vi "HDF5_Write_UPS_Record.vi"(0 "HealthRefs":T2 {"TimeStamp_dset" format="%.0x"; "TimeString_dset" format="%.0x"; "%_dset" format="%.0x"; "W_dset" format="%.0x"; "Hz_dset" format="%.0x"; "A_dset" format="%.0x"; "V_dset" format="%.0x"; "Group_ref" format="%.0x"}, 7 "UPS":T1, 11 "error in":errorcluster) -> (15 "error out":errorcluster)   [LabVIEW 2018]
doc: "Write a single Noise<x> record with timestamp:\nNoise1\n NoiseInfo - cluster with Timestamp and other metadata for this record\n SummdSpectrum - 1024 element Double array (waveform)"
uses:
  <vilib>/addons/h5labview2/dataset/H5D.lvlib
  <vilib>/addons/h5labview2/dataset/H5Dwrite.llb/H5Dwrite.xnode
  <vilib>/addons/h5labview2/space/H5S.lvlib
  <vilib>/addons/h5labview2/base/H5Equery.vi
  <vilib>/addons/h5labview2/base/lib_path.vi
  <vilib>/addons/h5labview2/base/hid_t_renamed.ctl
  UPS_refs.ctl
  Controls/Clusts/UPS_Status_Clust.ctl
  <vilib>/addons/h5labview2/base/hid_t.ctl
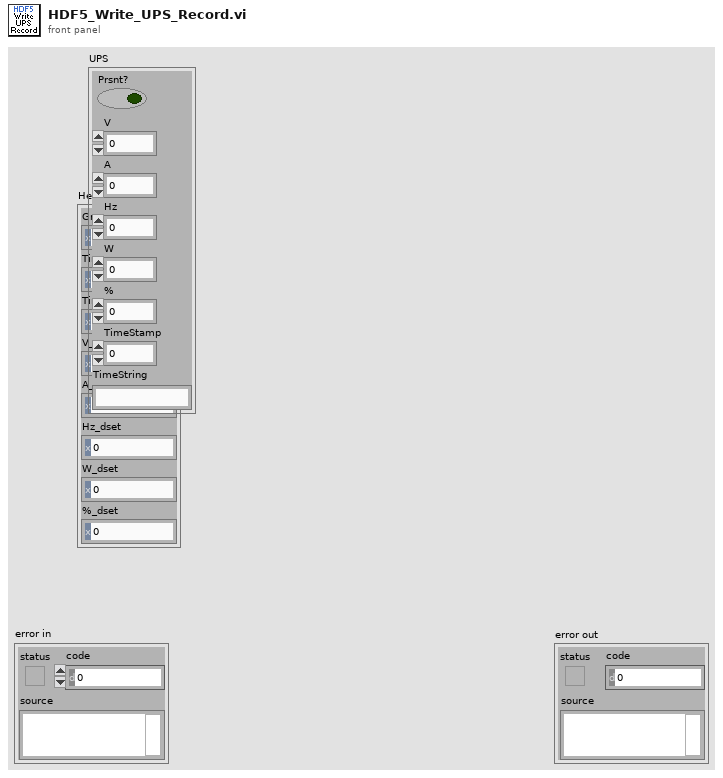
[diagram p1: front panel]
types:
  T1 = typedef "UPS_Status_Clust.ctl" = cluster{"Prsnt?":bool, "V":dbl, "A":dbl, "Hz":dbl, "W":dbl, "%":dbl, "TimeStamp":dbl, "TimeString":string}
  T2 = typedef "UPS_refs.ctl" = cluster{"Group_ref":T3, "TimeString_dset":T3, "TimeStamp_dset":T3, "V_dset":T3, "A_dset":T3, "Hz_dset":T3, "W_dset":T3, "%_dset":T3}
  T3 = typedef "hid_t.ctl" = i32
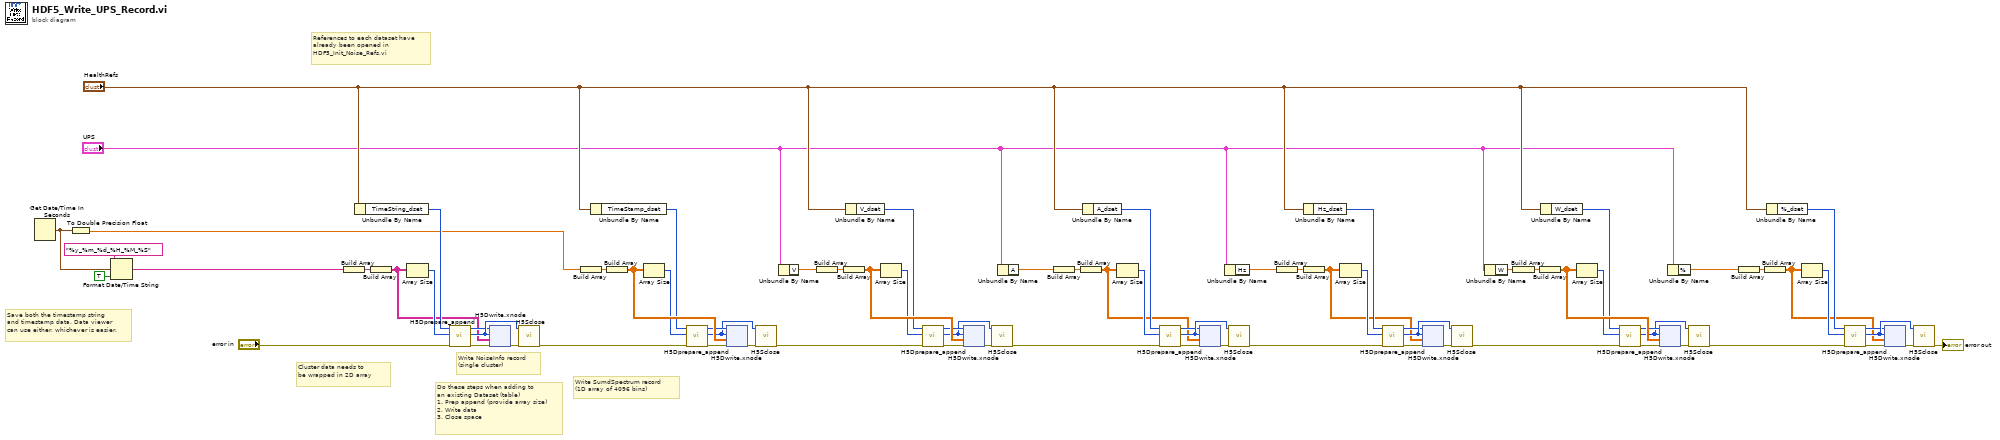
[diagram p0: block diagram]
diagram:
  # "Save both the timestamp string\nand timestamp data. Data viewer\ncan use either, whichever is easier."
  # "Cluster data needs to \nbe wrapped in 2D array"
  # "References to each dataset have \nalready been opened in \nHDF5_Init_Noise_Refs.vi"
  # "Do these steps when adding to \nan existing Dataset (table)\n1. Prep append (provide array size)\n2. Write data\n3. Close space"
  # "Write SumdSpectrum record\n(1D array of 4096 bins)"
  # "Write NoiseInfo record\n(single cluster)"
  n1 = Get Date/Time In Seconds() -> (seconds since 1Jan1904=w67:timestamp)
  n2 = To Double Precision Float(number=w67) -> (double precision float=w55:dbl)
  n3 = Format Date/Time String(time format string (%c)="%y_%m_%d_%H_%M_%S", seconds (now)=w67, UTC format=TRUE) -> (date/time string=w64:string)
  n4 = Build Array(w64) -> (w71:string[])
  n5 = Unbundle By Name("HealthRefs") -> ("TimeString_dset"=w70:T3)
  n6 = Build Array(w71) -> (w66:string[][])
  n7 = Array Size(array=w66) -> (size(s)=w69:i32[])
  n8 = call <vilib>:"H5Dprepare_append.vi"("error in (no error)"="error in", "append dims"=w69, "dset in"=w70) -> ("error out"=w76:errorcluster, "space out"=w74:T3, "dset out"=w73:T3)  [unwired: 5 in, 1 out]
  n9 = xnode "H5Dwrite.xnode"("error in (no error)"=w76, "data"=w66, "file space"=w74, "ref in"=w73) -> ("error out"=w75:errorcluster)  [unwired: 3 in, 2 out]
  n10 = call <vilib>:"H5Sclose.vi"("error in (no error)"=w75, "space in"=w74) -> ("error out"=w54:errorcluster)  [unwired: 9 in]
  n11 = Build Array(w55) -> (w60:dbl[])
  n12 = Unbundle By Name("HealthRefs") -> ("TimeStamp_dset"=w61:T3)
  n13 = Build Array(w60) -> (w63:dbl[][])
  n14 = Array Size(array=w63) -> (size(s)=w62:i32[])
  n15 = call <vilib>:"H5Dprepare_append.vi"("error in (no error)"=w54, "append dims"=w62, "dset in"=w61) -> ("error out"=w56:errorcluster, "space out"=w58:T3, "dset out"=w59:T3)  [unwired: 5 in, 1 out]
  n16 = xnode "H5Dwrite.xnode"("error in (no error)"=w56, "data"=w63, "file space"=w58, "ref in"=w59) -> ("error out"=w57:errorcluster)  [unwired: 3 in, 2 out]
  n17 = call <vilib>:"H5Sclose.vi"("error in (no error)"=w57, "space in"=w58) -> ("error out"=w9:errorcluster)  [unwired: 9 in]
  n18 = Unbundle By Name("UPS") -> ("V"=w7:dbl)
  n19 = Build Array(w7) -> (w41:dbl[])
  n20 = Build Array(w41) -> (w44:dbl[][])
  n21 = Unbundle By Name("HealthRefs") -> ("V_dset"=w42:T3)
  n22 = Array Size(array=w44) -> (size(s)=w43:i32[])
  n23 = call <vilib>:"H5Dprepare_append.vi"("error in (no error)"=w9, "append dims"=w43, "dset in"=w42) -> ("error out"=w37:errorcluster, "space out"=w39:T3, "dset out"=w40:T3)  [unwired: 5 in, 1 out]
  n24 = xnode "H5Dwrite.xnode"("error in (no error)"=w37, "data"=w44, "file space"=w39, "ref in"=w40) -> ("error out"=w38:errorcluster)  [unwired: 3 in, 2 out]
  n25 = call <vilib>:"H5Sclose.vi"("error in (no error)"=w38, "space in"=w39) -> ("error out"=w53:errorcluster)  [unwired: 9 in]
  n26 = Unbundle By Name("UPS") -> ("A"=w6:dbl)
  n27 = Build Array(w6) -> (w48:dbl[])
  n28 = Build Array(w48) -> (w45:dbl[][])
  n29 = Unbundle By Name("HealthRefs") -> ("A_dset"=w47:T3)
  n30 = Array Size(array=w45) -> (size(s)=w46:i32[])
  n31 = call <vilib>:"H5Dprepare_append.vi"("error in (no error)"=w53, "append dims"=w46, "dset in"=w47) -> ("error out"=w52:errorcluster, "space out"=w50:T3, "dset out"=w49:T3)  [unwired: 5 in, 1 out]
  n32 = xnode "H5Dwrite.xnode"("error in (no error)"=w52, "data"=w45, "file space"=w50, "ref in"=w49) -> ("error out"=w51:errorcluster)  [unwired: 3 in, 2 out]
  n33 = Unbundle By Name("UPS") -> ("Hz"=w5:dbl)
  n34 = call <vilib>:"H5Sclose.vi"("error in (no error)"=w51, "space in"=w50) -> ("error out"=w10:errorcluster)  [unwired: 9 in]
  n35 = Build Array(w5) -> (w32:dbl[])
  n36 = Unbundle By Name("HealthRefs") -> ("Hz_dset"=w31:T3)
  n37 = Build Array(w32) -> (w29:dbl[][])
  n38 = Array Size(array=w29) -> (size(s)=w30:i32[])
  n39 = call <vilib>:"H5Dprepare_append.vi"("error in (no error)"=w10, "append dims"=w30, "dset in"=w31) -> ("error out"=w36:errorcluster, "space out"=w34:T3, "dset out"=w33:T3)  [unwired: 5 in, 1 out]
  n40 = xnode "H5Dwrite.xnode"("error in (no error)"=w36, "data"=w29, "file space"=w34, "ref in"=w33) -> ("error out"=w35:errorcluster)  [unwired: 3 in, 2 out]
  n41 = call <vilib>:"H5Sclose.vi"("error in (no error)"=w35, "space in"=w34) -> ("error out"=w20:errorcluster)  [unwired: 9 in]
  n42 = Unbundle By Name("UPS") -> ("W"=w2:dbl)
  n43 = Build Array(w2) -> (w25:dbl[])
  n44 = Build Array(w25) -> (w28:dbl[][])
  n45 = Unbundle By Name("HealthRefs") -> ("W_dset"=w26:T3)
  n46 = Array Size(array=w28) -> (size(s)=w27:i32[])
  n47 = call <vilib>:"H5Dprepare_append.vi"("error in (no error)"=w20, "append dims"=w27, "dset in"=w26) -> ("error out"=w21:errorcluster, "space out"=w23:T3, "dset out"=w24:T3)  [unwired: 5 in, 1 out]
  n48 = xnode "H5Dwrite.xnode"("error in (no error)"=w21, "data"=w28, "file space"=w23, "ref in"=w24) -> ("error out"=w22:errorcluster)  [unwired: 3 in, 2 out]
  n49 = Unbundle By Name("UPS") -> ("%"=w1:dbl)
  n50 = call <vilib>:"H5Sclose.vi"("error in (no error)"=w22, "space in"=w23) -> ("error out"=w11:errorcluster)  [unwired: 9 in]
  n51 = Build Array(w1) -> (w15:dbl[])
  n52 = Build Array(w15) -> (w12:dbl[][])
  n53 = Unbundle By Name("HealthRefs") -> ("%_dset"=w14:T3)
  n54 = Array Size(array=w12) -> (size(s)=w13:i32[])
  n55 = call <vilib>:"H5Dprepare_append.vi"("error in (no error)"=w11, "append dims"=w13, "dset in"=w14) -> ("error out"=w19:errorcluster, "space out"=w17:T3, "dset out"=w16:T3)  [unwired: 5 in, 1 out]
  n56 = xnode "H5Dwrite.xnode"("error in (no error)"=w19, "data"=w12, "file space"=w17, "ref in"=w16) -> ("error out"=w18:errorcluster)  [unwired: 3 in, 2 out]
  n57 = call <vilib>:"H5Sclose.vi"("error in (no error)"=w18, "space in"=w17) -> ("error out"=→"error out":errorcluster)  [unwired: 9 in]
